vi "y_axis_pid_v4.vi"(10 "PID Gains":T1={"Proportional Gain (Kc)"=0.8, "Integral Gain"=25.0, "Derivative Gain"=0.004}, 11 "Y In":dbl=-1.0 format="%.3f") -> (0 "Motor 4":dbl, 1 "Motor 3":dbl, 2 "Motor 2":dbl, 3 "Motor 1":dbl, 4 "error out":errorcluster)   [LabVIEW 2019]
uses:
  <vilib>/addons/control/pid/pid.llb/PID (DBL).vi
  <vilib>/addons/control/pid/NI_PID_pid.lvlib
panel:
  out "PID Out":dbl=1.8829840965238862 format="%0#4.1g"
  in  "Reinitialize":bool
  in  "stop":bool
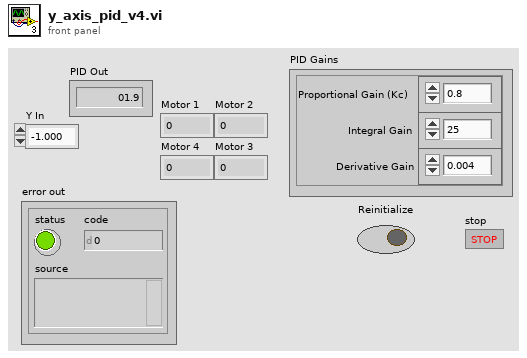
[diagram p1: front panel]
types:
  T1 = cluster{"Proportional Gain (Kc)":dbl, "Integral Gain":dbl, "Derivative Gain":dbl}
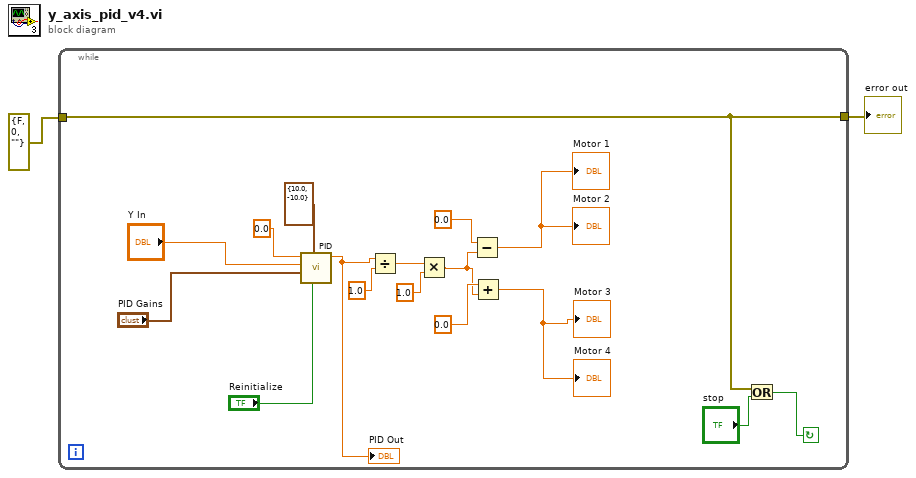
[diagram p0: block diagram]
diagram:
  n1 = while {
    tunnel: errorcluster {"status"=FALSE, "code"=0, "source"=""} ("error in (no error)") -> [w12]
    tunnel: [w12] -> w1
    stop <- w13 continue-if-true
    n2 = call-poly <vilib>:"PID.vi"("reinitialize? (F)"="Reinitialize", "output range"=cluster{"output high":dbl, "output low":dbl} {"output high"=10.0, "output low"=-10.0}, "PID gains"="PID Gains", "process variable"="Y In", "setpoint"=0.0 ("Angle (rads)")) -> ("output"=w6:dbl)  [unwired: 5 in, 1 out]
    "PID Out" <- w6
    n3 = Divide(x=w6, y=1.0) -> (x/y=w9:dbl)
    n4 = Multiply(x=w9, y=1.0) -> (x*y=w5:dbl)
    n5 = Subtract(x=0.0, y=w5) -> (x-y=→"Motor 1" →"Motor 2":dbl)
    n6 = Add(x=0.0, y=w5) -> (x+y=→"Motor 4" →"Motor 3":dbl)
    n7 = Or(x=w12, y="stop") -> (x .or. y?=w13:bool)
  }
  "error out" <- w1
